vi "Calculate Power Spectrum.vi"(0 "IQ data":cdb[](array[numeric]), 5 "sample rate":dbl) -> (4 "power spectrum (dBm)":cluster{"f0":dbl, "df":dbl, "magnitude":dbl[]})   [LabVIEW 2015]
doc: "Calculates the power spectrum from the I/Q waveform."
uses:
  <vilib>/measure/maspectr.llb/FFT Power Spectrum and PSD for 1 Chan (CDB).vi
  <vilib>/measure/NI_MAPro.lvlib
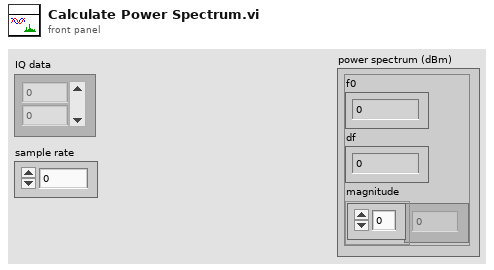
[diagram p1: front panel]
types:
  T1 = cluster{"averaging mode":enum16{"No averaging", "Vector averaging", "RMS averaging", "Peak hold"}, "weighting mode":enum16{"Linear", "Exponential"}, "number of averages":u32}
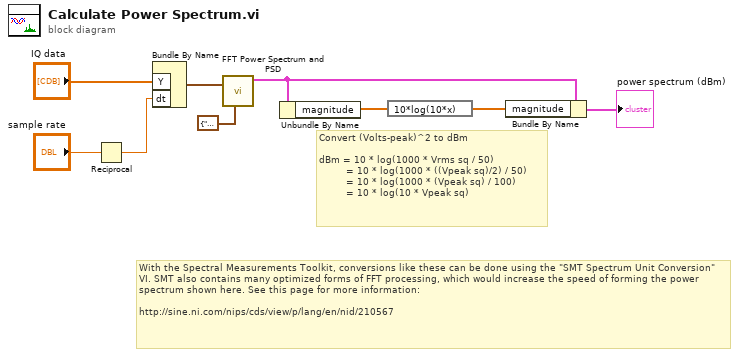
[diagram p0: block diagram]
diagram:
  # "With the Spectral Measurements Toolkit, conversions like these can be done using the \"SMT Spectrum Unit Conversion\" VI. SMT also contains many optimized forms of FFT processing, which would increase the speed of forming the power spectrum shown here. See this page for more information: \n\nhttp://sine.ni.com/nips/cds/view/p/lang/en/nid/210567"
  # "Convert (Volts-peak)^2 to dBm\n\ndBm = 10 * log(1000 * Vrms sq / 50)\n         = 10 * log(1000 * ((Vpeak sq)/2) / 50) \n         = 10 * log(1000 * (Vpeak sq) / 100) \n         = 10 * log(10 * Vpeak sq)"
  n1 = Reciprocal(x="sample rate") -> (1/x=w2:dbl)
  n2 = Bundle By Name("Y"="IQ data", "dt"=w2) -> (w3:waveform(cdb))  [unwired: 1 in]
  n3 = call-poly <vilib>:"FFT Power Spectrum and PSD.vi"("averaging parameters"=T1 {"averaging mode"=enum."No averaging", "weighting mode"=enum."Exponential", "number of averages"=10}, "time signal"=w3) -> ("Power Spectrum / PSD"=w7:cluster{"f0":dbl, "df":dbl, "magnitude":dbl[]})  [unwired: 6 in, 3 out]
  n4 = Unbundle By Name(w7) -> ("magnitude"=w8:dbl[])
  n5 = expression code="10*log(10*x)"(w8) -> (w9:dbl[])
  n6 = Bundle By Name(cluster=w7, "magnitude"=w9) -> (→"power spectrum (dBm)":cluster{"f0":dbl, "df":dbl, "magnitude":dbl[]})
